vi "test_header_map.vi"() -> ()   [LabVIEW 2020, in "reqwest_tests.lvlib"]
uses:
  reqwest_tests.lvlib
  Headers/Headers.lvclass
  <vilib>/addons/_JKI Toolkits/Caraya/classes/Assert/Assert.lvclass
  <vilib>/addons/_JKI Toolkits/Caraya/classes/Test/Test.lvclass
panel:
  out "success":bool
  in  "error in (no error)":errorcluster
  out "error out":errorcluster
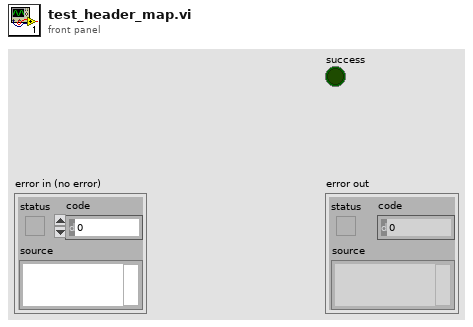
[diagram p1: front panel]
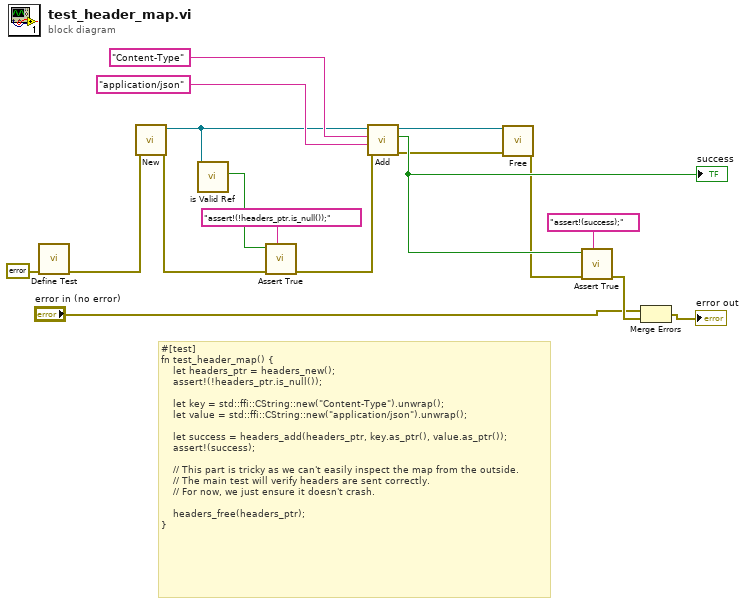
[diagram p0: block diagram]
diagram:
  # "#[test]\nfn test_header_map() {\n    let headers_ptr = headers_new();\n    assert!(!headers_ptr.is_null());\n\n    let key = std::ffi::CString::new(\"Content-Type\").unwrap();\n    let value = std::ffi::CString::new(\"application/json\").unwrap();\n\n    let success = headers_add(headers_ptr, key.as_ptr(), value.as_ptr());\n    assert!(success);\n\n    // This part is tricky as we can't easily inspect the map from the outside.\n    // The main test will verify headers are sent correctly.\n    // For now, we just ensure it doesn't crash.\n\n    headers_free(headers_ptr);\n}"
  n1 = call <vilib>:"Define Test.vi"("error in (no error)"=errorcluster {"status"=FALSE, "code"=0, "source"=""}) -> ("error out"=w7:errorcluster)  [unwired: 9 in, 1 out]
  n2 = call "New.vi"("error in (no error)"=w7) -> ("error out"=w2:errorcluster, "Headers out"=w5:refnum<class "Headers.lvclass">)  [unwired: 9 in]
  n3 = call "is Valid Ref.vi"("Headers in"=w5) -> ("valid-ref?"=w3:bool)  [unwired: 10 in]
  n4 = call <vilib>:"Assert True.vi"("Label"="assert!(!headers_ptr.is_null());", "error in (no error)"=w2, "True?"=w3) -> ("error out"=w1:errorcluster)  [unwired: 7 in, 1 out]
  n5 = call "Add.vi"("error in (no error)"=w1, "value"="application/json", "key"="Content-Type", "Headers in"=w5) -> ("error out"=w15:errorcluster, "success"=w16:bool, "Headers out"=w17:refnum<class "Headers.lvclass">)  [unwired: 5 in]
  "success" <- w16
  n6 = call "Free.vi"("error in (no error)"=w15, "Headers in"=w17) -> ("error out"=w14:errorcluster)  [unwired: 9 in]
  n7 = call <vilib>:"Assert True.vi"("Label"="assert!(success);", "error in (no error)"=w14, "True?"=w16) -> ("error out"=w13:errorcluster)  [unwired: 7 in, 1 out]
  n8 = Merge Errors("error in (no error)", w13) -> (→"error out":errorcluster)
